vi "NF87XX.separate numeric Driver Infos.vi"(1 "Driver":string, 2 "Read String":string) -> (16 "Result":dbl[](array[numeric]))   [LabVIEW 2014, in "NF87XX.lvlib"]
doc: "This VI sorts information of a NF device according to the device syntax."
uses:
  NF87XX.lvlib
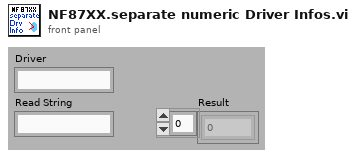
[diagram p1: front panel]
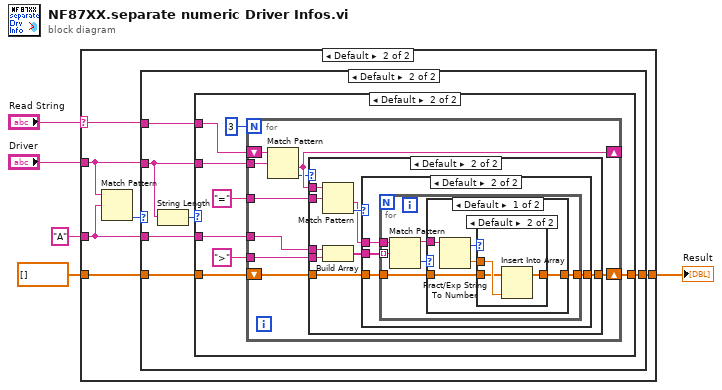
[diagram p0: block diagram]
diagram:
  n1 = case shown="Default" "Read String" {
    selector: "Read String" -> [_ w12]
    tunnel: "Driver" -> [_ w9]
    tunnel: [w6 w11] -> w3
    tunnel: dbl[] [] -> [w6 w10]
    tunnel: "A" ("regular expression") -> [_ w8]
    frame "" {
    }
    frame Default {
      n2 = Match Pattern(string=w9, regular expression=w8) -> (offset past match=w7:i32)  [unwired: 1 in, 3 out]
      n3 = case shown="Default" w7 {
        tunnel: w12 -> [_ w19]
        tunnel: [w13 w18] -> w11
        tunnel: w10 -> [w13 w17]
        tunnel: w8 -> [_ w16]
        tunnel: w9 -> [_ w14]
        frame -1 {
        }
        frame Default {
          n4 = String Length(string=w14) -> (length=w15:i32)
          n5 = case shown="Default" w15 {
            tunnel: w19 -> [_ w25]
            tunnel: [w20 w24] -> w18
            tunnel: w17 -> [w20 w23]
            tunnel: w14 -> [_ w22]
            tunnel: w16 -> [_ w21]
            frame 0, 1 {
            }
            frame Default {
              n6 = for {
                N: 3 -> [_]
                tunnel: w22 -> [w36]
                shift-right: [w35] -> _
                shift-left: w25 -> [w37]
                tunnel: "=" ("regular expression") -> [w33]
                tunnel: ">" ("regular expression") -> [w31]
                tunnel: w21 -> [w32]
                shift-right: [w30] -> w24
                shift-left: w23 -> [w29]
                n7 = Match Pattern(string=w37, regular expression=w36) -> (after substring=w35:string, offset past match=w34:i32)  [unwired: 1 in, 2 out]
                n8 = case shown="Default" w34 {
                  tunnel: w35 -> [_ w47]
                  tunnel: w33 -> [_ w46]
                  tunnel: w31 -> [_ w42]
                  tunnel: w32 -> [_ w43]
                  tunnel: [w38 w40] -> w30
                  tunnel: w29 -> [w38 w39]
                  frame -1 {
                  }
                  frame Default {
                    n9 = Match Pattern(string=w47, regular expression=w46) -> (after substring=w44:string, offset past match=w45:i32)  [unwired: 1 in, 2 out]
                    n10 = Build Array(w43, w42) -> (w41:string[])
                    n11 = case shown="Default" w45 {
                      tunnel: w44 -> [_ w52]
                      tunnel: w41 -> [_ w51]
                      tunnel: [w48 w50] -> w40
                      tunnel: w39 -> [w48 w49]
                      frame -1 {
                      }
                      frame Default {
                        n12 = for {
                          tunnel: w52 -> [w58]
                          tunnel: w51 -> [w57] mode=indexing
                          tunnel: [w54] -> w50
                          tunnel: w49 -> [w53]
                          n13 = Match Pattern(string=w58, regular expression=w57) -> (before substring=w55:string, offset past match=w56:i32)  [unwired: 1 in, 2 out]
                          n14 = case shown="Default" w56 {
                            tunnel: w55 -> [w63 _]
                            tunnel: [w60 w68] -> w54
                            tunnel: w53 -> [w59 w68]
                            frame Default {
                              n15 = Fract/Exp String To Number(string=w63) -> (offset past number=w62:i32, number=w61:dbl)  [unwired: 3 in]
                              n16 = case shown="Default" w62 {
                                tunnel: w61 -> [_ w67]
                                tunnel: [w64 w66] -> w60
                                tunnel: w59 -> [w64 w65]
                                frame 0 {
                                }
                                frame Default {
                                n17 = Insert Into Array(array=w65, new element=w67) -> (w66:dbl[])  [unwired: 1 in]
                                }
                              }
                            }
                            frame -1 {
                            }
                          }
                        }
                      }
                    }
                  }
                }
              }
            }
          }
        }
      }
    }
  }
  "Result" <- w3
